vi "Load Parameters From XML.vi"() -> (4 "kinematic parameters":T6, 6 "dynamic parameters":cluster{"Thumb":T3, "Middle":T3, "Index":T3}, 8 "motor parameters":T2, 10 "finger offsets":T1, 15 "error out":errorcluster)   [LabVIEW 2011, in "MF3.lvclass"]
uses:
  MF3.lvclass
  <vilib>/robotics/Kinematics/Link/Joint Type.ctl
  controls/5-bar Side.ctl
  controls/Dynamic Parameters.ctl
  <vilib>/NI/GXML/_subVIs/GXML SearchParser/Search Parser.vi
  <vilib>/NI/GXML/GXML.lvlib
  <vilib>/robotics/Kinematics/Link/NI_Robotics_Link.lvclass
panel:
  out "file path":path
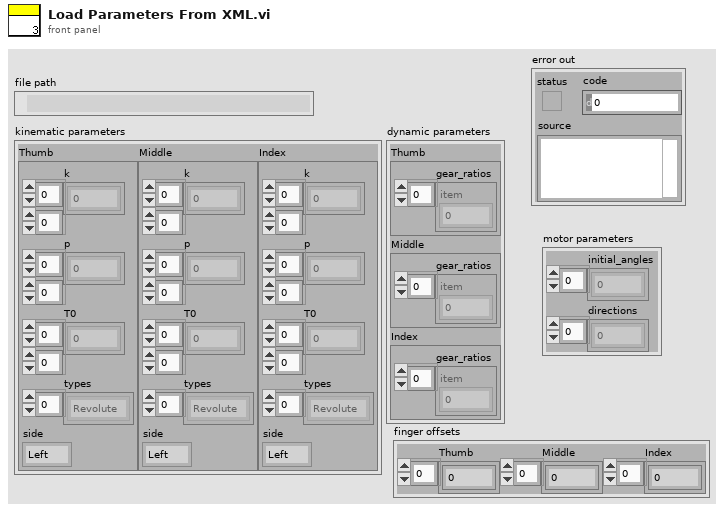
[diagram p1: front panel]
types:
  T1 = cluster{"Thumb":dbl[], "Middle":dbl[], "Index":dbl[]}
  T2 = cluster{"initial_angles":sgl[], "directions":sgl[]}
  T3 = typedef "Dynamic Parameters.ctl" = cluster{"gear_ratios":sgl[]}
  T4 = typedef "NI_Robotics_Link.lvclass/Joint Type.ctl" = enum16{"Revolute", "Prismatic"}
  T5 = typedef "5-bar Side.ctl" = enum16{"Left", "Right"}
  T6 = cluster{"Thumb":cluster{"k":sgl[][], "p":sgl[][], "T0":sgl[][], "types":T4[], "side":T5}, "Middle":cluster{"k":sgl[][], "p":sgl[][], "T0":sgl[][], "types":T4[], "side":T5}, "Index":cluster{"k":sgl[][], "p":sgl[][], "T0":sgl[][], "types":T4[], "side":T5}}
  T7 = cluster{"Thumb":sgl[], "Middle":sgl[], "Index":sgl[]}
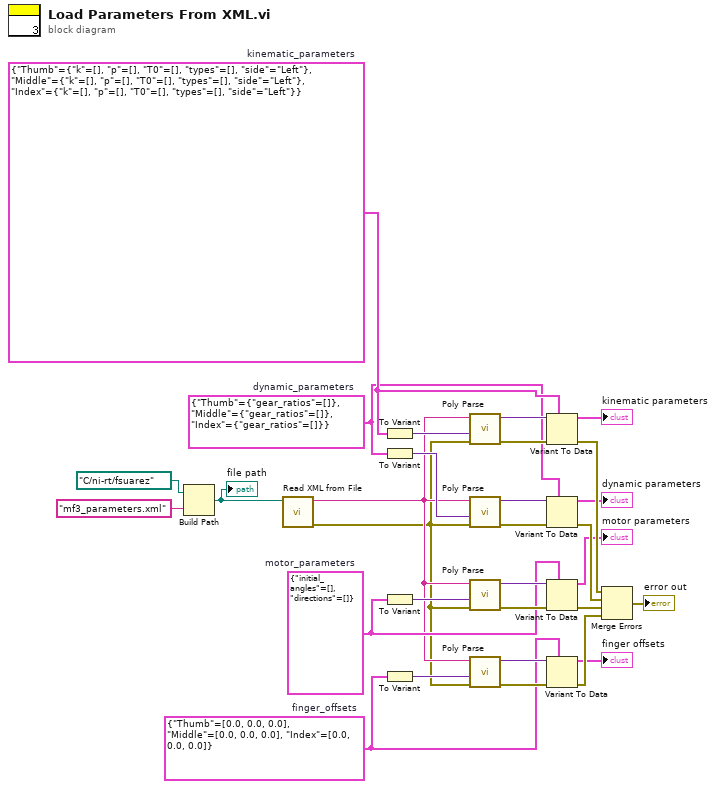
[diagram p0: block diagram]
diagram:
  w4 = T7 {"Thumb"=[0.0, 0.0, 0.0], "Middle"=[0.0, 0.0, 0.0], "Index"=[0.0, 0.0, 0.0]}  # finger_offsets
  w11 = T2 {"initial_angles"=[], "directions"=[]}  # motor_parameters
  w20 = cluster{"Thumb":T3, "Middle":T3, "Index":T3} {"Thumb"={"gear_ratios"=[]}, "Middle"={"gear_ratios"=[]}, "Index"={"gear_ratios"=[]}}  # dynamic_parameters
  w25 = T6 {"Thumb"={"k"=[], "p"=[], "T0"=[], "types"=[], "side"=enum."Left"}, "Middle"={"k"=[], "p"=[], "T0"=[], "types"=[], "side"=enum."Left"}, "Index"={"k"=[], "p"=[], "T0"=[], "types"=[], "side"=enum."Left"}}  # kinematic_parameters
  n1 = Build Path(base path=path "C:/ni-rt/fsuarez", name or relative path="mf3_parameters.xml") -> (appended path=w28:path)
  "file path" <- w28
  n2 = call <vilib>:"Read XML from File.vi"("XML File Path"=w28) -> ("error out"=w2:errorcluster, "XML String Out"=w6:string)  [unwired: 9 in]
  n3 = To Variant(anything=w25) -> (Variant=w27:variant)
  n4 = To Variant(anything=w20) -> (Variant=w23:variant)
  n5 = To Variant(anything=w11) -> (Variant=w12:variant)
  n6 = To Variant(anything=w4) -> (Variant=w5:variant)
  n7 = call-poly <vilib>:"Poly Parse.vi"("error in"=w2, "TypeDesc"=w27, "XML String In"=w6) -> ("error out"=w22:errorcluster, "Parsed Data"=w26:variant)  [unwired: 7 in]
  n8 = call-poly <vilib>:"Poly Parse.vi"("error in"=w2, "TypeDesc"=w23, "XML String In"=w6) -> ("error out"=w18:errorcluster, "Parsed Data"=w19:variant)  [unwired: 7 in]
  n9 = call-poly <vilib>:"Poly Parse.vi"("error in"=w2, "TypeDesc"=w12, "XML String In"=w6) -> ("error out"=w13:errorcluster, "Parsed Data"=w14:variant)  [unwired: 7 in]
  n10 = call-poly <vilib>:"Poly Parse.vi"("error in"=w2, "TypeDesc"=w5, "XML String In"=w6) -> ("error out"=w7:errorcluster, "Parsed Data"=w8:variant)  [unwired: 7 in]
  n11 = Variant To Data(error in=w22, type=w25, Variant=w26) -> (data=→"kinematic parameters":T6, error out=w21:errorcluster)
  n12 = Variant To Data(error in=w18, type=w20, Variant=w19) -> (data=→"dynamic parameters":cluster{"Thumb":T3, "Middle":T3, "Index":T3}, error out=w17:errorcluster)
  n13 = Variant To Data(error in=w13, type=w11, Variant=w14) -> (data=→"motor parameters":T2, error out=w9:errorcluster)
  n14 = Variant To Data(error in=w7, type=w4, Variant=w8) -> (data=→"finger offsets":T7, error out=w3:errorcluster)
  n15 = Merge Errors(w21, w17, w9, w3) -> (→"error out":errorcluster)
